vi "Read Elastic Moduli Configuration.vi"(8 "error in (no error)":errorcluster, 11 "Elastic Moduli in":refnum<class "Format Resonances.lvclass">) -> (0 "error out":errorcluster, 2 "Configuration":T1, 3 "Elastic Moduli out":refnum<class "Format Resonances.lvclass">)   [LabVIEW 2018, in "Format Resonances.lvclass"]
uses:
  Format Resonances.lvclass
  C:/github/2018/LabActor/Template Module/Template Module.lvclass
  Format Resonances Configuration.ctl
  Template Module/Template Module.lvclass/Template Module.ctl
  Template Module/Read Configuration.vi
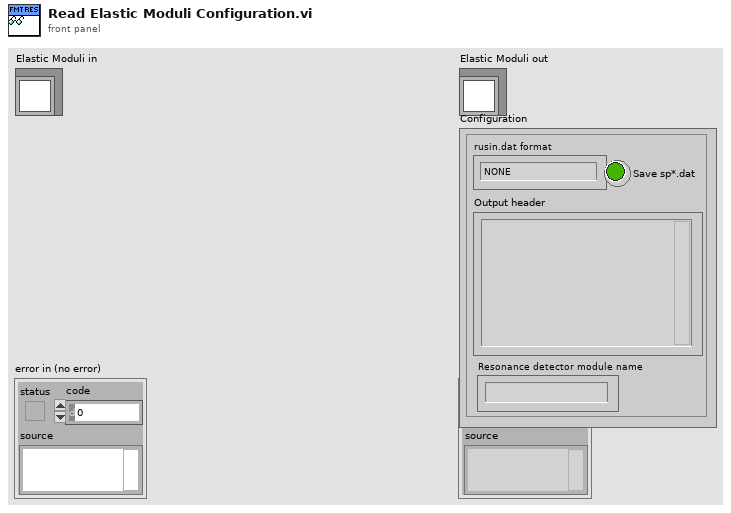
[diagram p1: front panel]
types:
  T1 = typedef "Format Resonances Configuration.ctl" = cluster{"Output header ":string, "rusin\n.dat":enum16{"NONE", "With header", "Without header"}, "Resonance detector module name":string, "Save sp*.dat":bool}
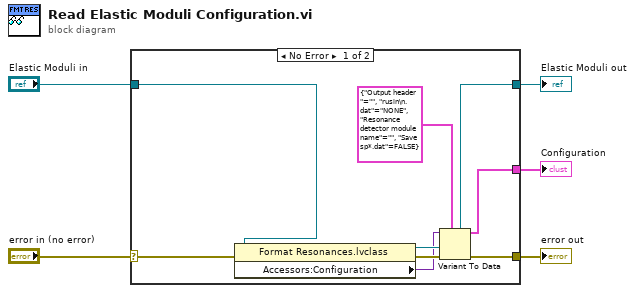
[diagram p0: block diagram]
diagram:
  n1 = case shown="No Error" "error in (no error)" {
    selector: "error in (no error)" -> [w13 w14]
    tunnel: [w9 w14] -> w4
    tunnel: [w10 w15] -> w2
    tunnel: "Elastic Moduli in" -> [w11 w15]
    tunnel: [w6 _] -> w1
    frame No Error {
      n2 = property class="Format Resonances.lvclass"(reference=w11, error in=w13) -> (reference out=w10:refnum<class "Format Resonances.lvclass">, error out=w12:errorcluster, "Accessors:Configuration"=w8:variant)
      n3 = Variant To Data(error in=w12, type=T1 {"Output header "="", "rusin\n.dat"=enum."NONE", "Resonance detector module name"="", "Save sp*.dat"=FALSE} ("Configuration"), Variant=w8) -> (data=w6:T1, error out=w9:errorcluster)
    }
    frame Error {
    }
  }
  "error out" <- w4
  "Elastic Moduli out" <- w2
  "Configuration" <- w1
